vi "Wire Is Different as WhileLoop EndRef Wire.vi"(11 "Wire in":refnum<vi>) -> (3 "is different than WhileLoop endref?":bool)   [LabVIEW 2014]
doc: "Return if wire is different than wire connected to WhileLoop. If wire is not even in structure it returns TRUE, because it is not in that case wired to end terminal of WhileLoop.\nUsed for wire declaration to not generate declaration for stop wire inside WhileLoop."
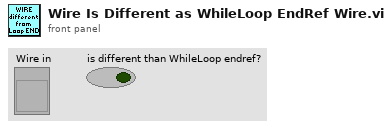
[diagram p1: front panel]
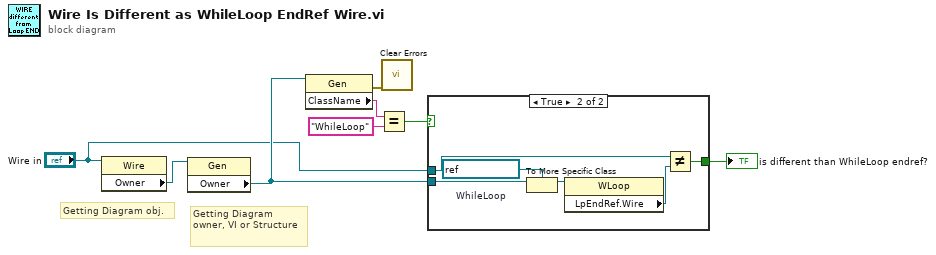
[diagram p0: block diagram]
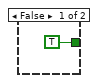
[diagram p2: hidden frame]
diagram:
  # "Getting Diagram owner, VI or Structure"
  # "Getting Diagram obj."
  n1 = property class="Wire"(reference="Wire in") -> ("Owner"=w3:refnum<vi>)  [unwired: 1 in, 2 out]
  n2 = property class="Gen"(reference=w3) -> ("Owner"=w2:refnum<vi>)  [unwired: 1 in, 2 out]
  n3 = property class="Gen"(reference=w2) -> (error out=w8:errorcluster, "ClassName"=w4:string)  [unwired: 1 in, 1 out]
  n4 = Equal?(x=w4, y="WhileLoop") -> (x = y?=w6:bool)
  n5 = call <vilib>:"Clear Errors.vi"("error in (no error)"=w8) -> ()  [unwired: 5 in, 2 out]
  n6 = case shown="True" w6 {
    tunnel: "Wire in" -> [_ w12]
    tunnel: [TRUE w11] -> w7
    tunnel: w2 -> [_ w10]
    frame False {
    }
    frame True {
      w15 = refnum<vi> refnum  # WhileLoop
      n7 = To More Specific Class(target class=w15, reference=w10) -> (specific class reference=w14:refnum<vi>)  [unwired: 1 in, 1 out]
      n8 = property class="WLoop"(reference=w14) -> ("LpEndRef.Wire"=w13:refnum<vi>)  [unwired: 1 in, 2 out]
      n9 = Not Equal?(x=w12, y=w13) -> (x != y?=w11:bool)
    }
  }
  "is different than WhileLoop endref?" <- w7
